vi "Run Test.vi"(8 "error in (no error)":errorcluster, 11 "LED Board Visual Test in":refnum<class "LED Board Test.lvclass">) -> (0 "error out":errorcluster, 1 "Positions":i32[](array[numeric]), 2 "Tests Passed":bool[](array[boolean]), 3 "LED Board Visual Test out":refnum<class "LED Board Test.lvclass">, 5 "Fail Codes":string[](array[string]))   [LabVIEW 2015, in "LED Board Test.lvclass"]
uses:
  LED Board Test.lvclass
  CBTF Applications/LED Board Testing/Main/Application/Application/Class/LED Board.lvclass
  LED Board Test.lvclass/LED Board Test.ctl
  Test Class/Test Class.lvclass
  Classes/Application/Class/Application.lvclass
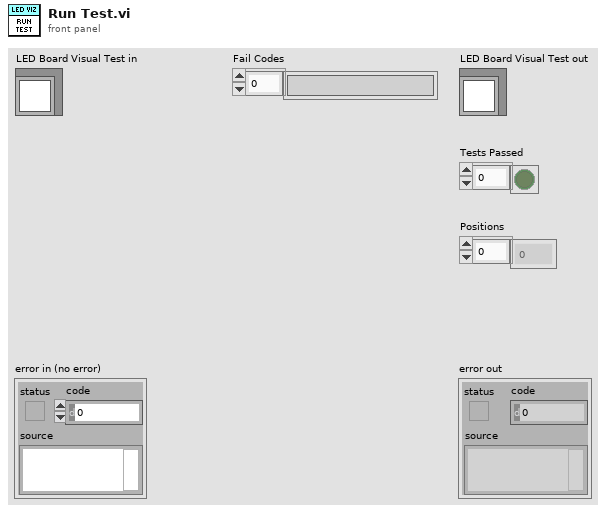
[diagram p1: front panel]
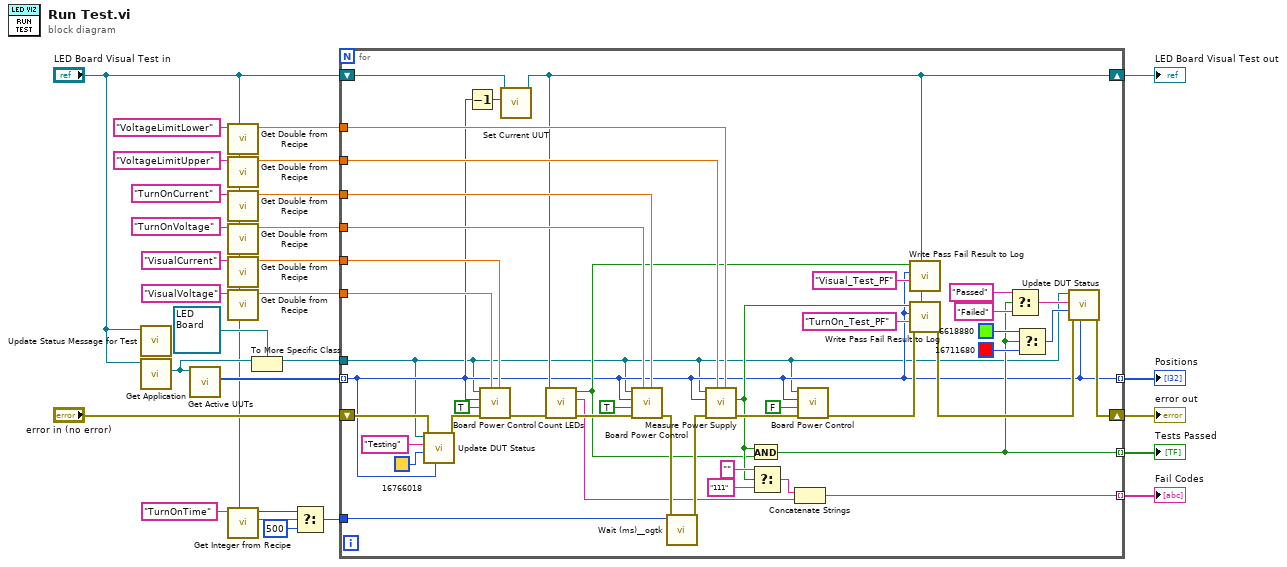
[diagram p0: block diagram]
diagram:
  n1 = call-dynamic "Update Status Message for Test.vi"("LED Board Power Test in"="LED Board Visual Test in") -> ()  [unwired: 11 in]
  n2 = call "Get Application.vi"("Test Class in"="LED Board Visual Test in") -> ("Application.lvlib:Application.lvclass"=w22:refnum<class "Application.lvclass">)  [unwired: 9 in, 1 out]
  n3 = call "Get Active UUTs.vi"("Application in"=w22) -> ("Active Positions"=w28:u32[])  [unwired: 8 in, 2 out]
  n4 = call "Get Double from Recipe.vi"("Test Class in"="LED Board Visual Test in", "Name"="VoltageLimitLower") -> ("Value"=w7:dbl)  [unwired: 7 in, 2 out]
  n5 = call "Get Double from Recipe.vi"("Test Class in"="LED Board Visual Test in", "Name"="VoltageLimitUpper") -> ("Value"=w8:dbl)  [unwired: 7 in, 2 out]
  n6 = call "Get Double from Recipe.vi"("Test Class in"="LED Board Visual Test in", "Name"="TurnOnCurrent") -> ("Value"=w9:dbl)  [unwired: 7 in, 2 out]
  n7 = call "Get Double from Recipe.vi"("Test Class in"="LED Board Visual Test in", "Name"="TurnOnVoltage") -> ("Value"=w10:dbl)  [unwired: 7 in, 2 out]
  n8 = call "Get Double from Recipe.vi"("Test Class in"="LED Board Visual Test in", "Name"="VisualCurrent") -> ("Value"=w11:dbl)  [unwired: 7 in, 2 out]
  n9 = call "Get Double from Recipe.vi"("Test Class in"="LED Board Visual Test in", "Name"="VisualVoltage") -> ("Value"=w12:dbl)  [unwired: 7 in, 2 out]
  n10 = call "Get Integer from Recipe.vi"("Test Class in"="LED Board Visual Test in", "Name"="TurnOnTime") -> ("found?"=w4:bool, "Value"=w5:i32)  [unwired: 7 in, 1 out]
  n11 = To More Specific Class(target class=refnum<class "LED Board.lvclass"> refnum ("LED Board.lvlib:LED Board.lvclass"), reference=w22) -> (specific class reference=w20:refnum<class "LED Board.lvclass">)  [unwired: 1 in, 1 out]
  n12 = Select(t=w5, s=w4, f=500) -> (s? t:f=w2:i32)
  n13 = for {
    shift-right: [w38] -> w23
    shift-left: "error in (no error)" -> [w40]
    shift-right: [w43] -> w24
    shift-left: "LED Board Visual Test in" -> [w68]
    tunnel: [w48] -> w25 mode=indexing
    tunnel: [w31] -> w26 mode=indexing
    tunnel: w28 -> [w30] mode=indexing
    tunnel: w12 -> [w63]
    tunnel: w11 -> [w64]
    tunnel: w20 -> [w29]
    tunnel: [w30] -> w19 mode=indexing
    tunnel: w10 -> [w60]
    tunnel: w9 -> [w59]
    tunnel: w8 -> [w57]
    tunnel: w7 -> [w56]
    tunnel: w2 -> [w54]
    n14 = call "Update DUT Status.vi"("Position"=w30, "error in (no error)"=w40, "BG Color"=u32 16766018, "Message ('')"="Testing", "Application in"=w29) -> ("error out"=w39:errorcluster)  [unwired: 5 in, 1 out]
    n15 = Decrement(x=w30) -> (x-1=w67:u32)
    n16 = call-dynamic "Board Power Control.vi"("Current Limit (0.0 Amps)"=w64, "Voltage (0.0 VDC)"=w63, "error in (no error)"=w39, "Enabled"=TRUE, "Position"=w30, "LED Board in"=w29) -> ("error out"=w66:errorcluster)  [unwired: 5 in]
    n17 = call "Set Current UUT.vi"("Current UUT"=w67, "LED Board Visual Test in"=w68) -> ("LED Board Visual Test out"=w43:refnum<class "LED Board Test.lvclass">)  [unwired: 8 in, 1 out]
    n18 = call "Count LEDs.vi"("error in (no error)"=w66, "LED Board Visual Test in"=w43) -> ("error out"=w65:errorcluster, "Fail Codes"=w53:string, "Tests Passed"=w44:bool)  [unwired: 7 in]
    n19 = call-dynamic "Board Power Control.vi"("Current Limit (0.0 Amps)"=w59, "Voltage (0.0 VDC)"=w60, "error in (no error)"=w65, "Enabled"=TRUE, "Position"=w30, "LED Board in"=w29) -> ("error out"=w58:errorcluster)  [unwired: 5 in]
    n20 = call <userlib>:"Wait (ms)__ogtk.vi"("error in (no error)"=w58, "milliseconds to wait"=w54) -> ("error out"=w55:errorcluster)  [unwired: 8 in, 1 out]
    n21 = call-dynamic "Measure Power Supply.vi"("Lower Limit"=w56, "Upper Limit"=w57, "error in (no error)"=w55, "UUT"=w30, "LED Board in"=w29) -> ("error out"=w69:errorcluster, "In Range?"=w47:bool)  [unwired: 5 in]
    n22 = And(x=w47, y=w44) -> (x .and. y?=w31:bool)
    n23 = Select(t="" ("string"), s=w47, f="111" ("string")) -> (s? t:f=w49:string)
    n24 = Concatenate Strings(w49, w53) -> (w48:string)
    n25 = call-dynamic "Board Power Control.vi"("error in (no error)"=w69, "Enabled"=FALSE, "Position"=w30, "LED Board in"=w29) -> ("error out"=w71:errorcluster)  [unwired: 7 in]
    n26 = call "Write Pass Fail Result to Log.vi"("Test Class in"=w43, "Label"="Visual_Test_PF" ("Test Name"), "Position"=w30, "Result"=w44) -> ()  [unwired: 7 in, 1 out]
    n27 = call "Write Pass Fail Result to Log.vi"("Test Class in"=w43, "error in (no error)"=w71, "Label"="TurnOn_Test_PF" ("Test Name"), "Position"=w30, "Result"=w47) -> ("error out"=w70:errorcluster)  [unwired: 6 in]
    n28 = Select(t="Passed", s=w31, f="Failed") -> (s? t:f=w33:string)
    n29 = Select(t=u32 6618880, s=w31, f=u32 16711680) -> (s? t:f=w32:u32)
    n30 = call "Update DUT Status.vi"("Position"=w30, "error in (no error)"=w70, "BG Color"=w32, "Message ('')"=w33, "Application in"=w29) -> ("error out"=w38:errorcluster)  [unwired: 5 in, 1 out]
  }
  "error out" <- w23
  "LED Board Visual Test out" <- w24
  "Tests Passed" <- w26
  "Fail Codes" <- w25
  "Positions" <- w19
